vi "Simple Measurement.vi"() -> ()   [LabVIEW 2019]
doc: "Demonstrates how to initialize the bridge, configure measurement parameters, and perform both single and continuous measurements."
uses:
  <vilib>/Utility/file.llb/Write To Spreadsheet File (string).vi
  Andeen-Hagerling 2700A.lvlib
panel:
  in  "Clear":bool
  out "loss graph data":dbl[](array[numeric])
  out "time graph data":timestamp[](array[timestamp])
  out "cap graph data":dbl[](array[numeric])
  out "Measurement Buffer":string[](array[string])
  in  "Save":bool
  in  "cancel measure":bool
  out "Interface Information:Interface Type":u16(ring)=1 items=["GPIB"=1, "VXI"=2, "GPIB-VXI"=3, "Serial"=4, "PXI"=5, "TCPIP"=6, "USB"=7, "FireWire"=9]
  out "V 2":string
  out "Hz 2":string
  out "Capacitance Graph":cluster{timestamp[], dbl[]}(graph)
  out "Loss Graph":cluster{timestamp[], dbl[]}(graph)
  in  "Continuous":bool
  out "bridge error":T1
  out "Bridge Status":string
  out "Error Message":string
  out "V":string
  out "Hz":string
  out "pF":string
  in  "units":i32(ring)=1 items=["NS"=1, "DS"=2, "KO"=3, "GO"=4, "JP"=5]
  out "Applied Voltage":dbl format="%#_10f"
  out "Firmware Revision:":string
  in  "Maximum Applied Voltage":dbl=15.0
  in  "Average\nExponent":i32=4
  in  "Bridge Frequency":dbl=1000.0
  in  "stop":bool
  out "greater than":string
  out "Loss":dbl format="%#_10f"
  out "Measurement Frequency":dbl format="%#_10f"
  out "Capacitance":dbl format="%#_10f"
  out "measurement results":T2 {"Loss" format="%#_10f"; "Capacitance" format="%#_10f"; "Frequency" format="%#_8f"}
  in  "Measure":bool
  # "AH2700A ULTRA-PRECISION CAPACITANCE BRIDGE"
  # "Measurement Parameters"
  # "Measurement Results"
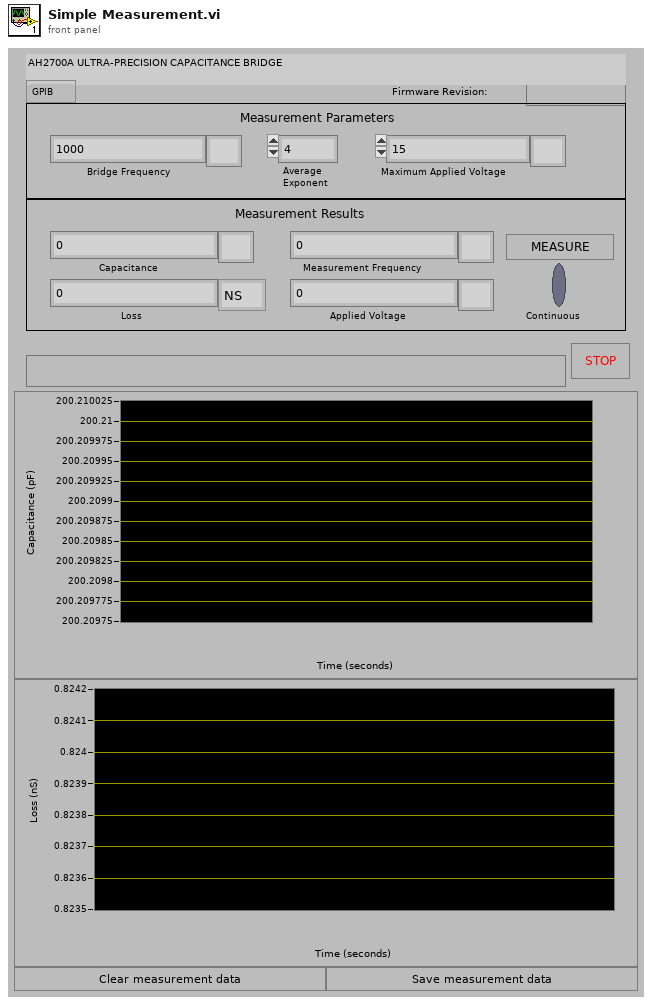
[diagram p1: front panel]
types:
  T1 = cluster{"error message":string, "error code":i32}
  T2 = cluster{"Error":i32, "Frequency":dbl, "Capacitance":dbl, "Loss":dbl, "GreaterThan":bool, "Voltage":dbl}
  T3 = cluster{"Baud Rate":u32, "Parity":u16, "Data Bits":u16, "Stop Bits":u16, "Flow Control":u16}
  T4 = cluster{"error":i32, "frequency":dbl, "capacitance":dbl, "loss":dbl, "greater than":bool, "voltage":dbl}
  T5 = cluster{"time graph data":timestamp[], "cap graph data":dbl[]}
  T6 = cluster{"time graph data":timestamp[], "loss graph data":dbl[]}
  T7 = cluster{"error code":i32, "frequency":dbl, "capacitance":dbl, "loss":dbl, "greater than":bool, "voltage":dbl}
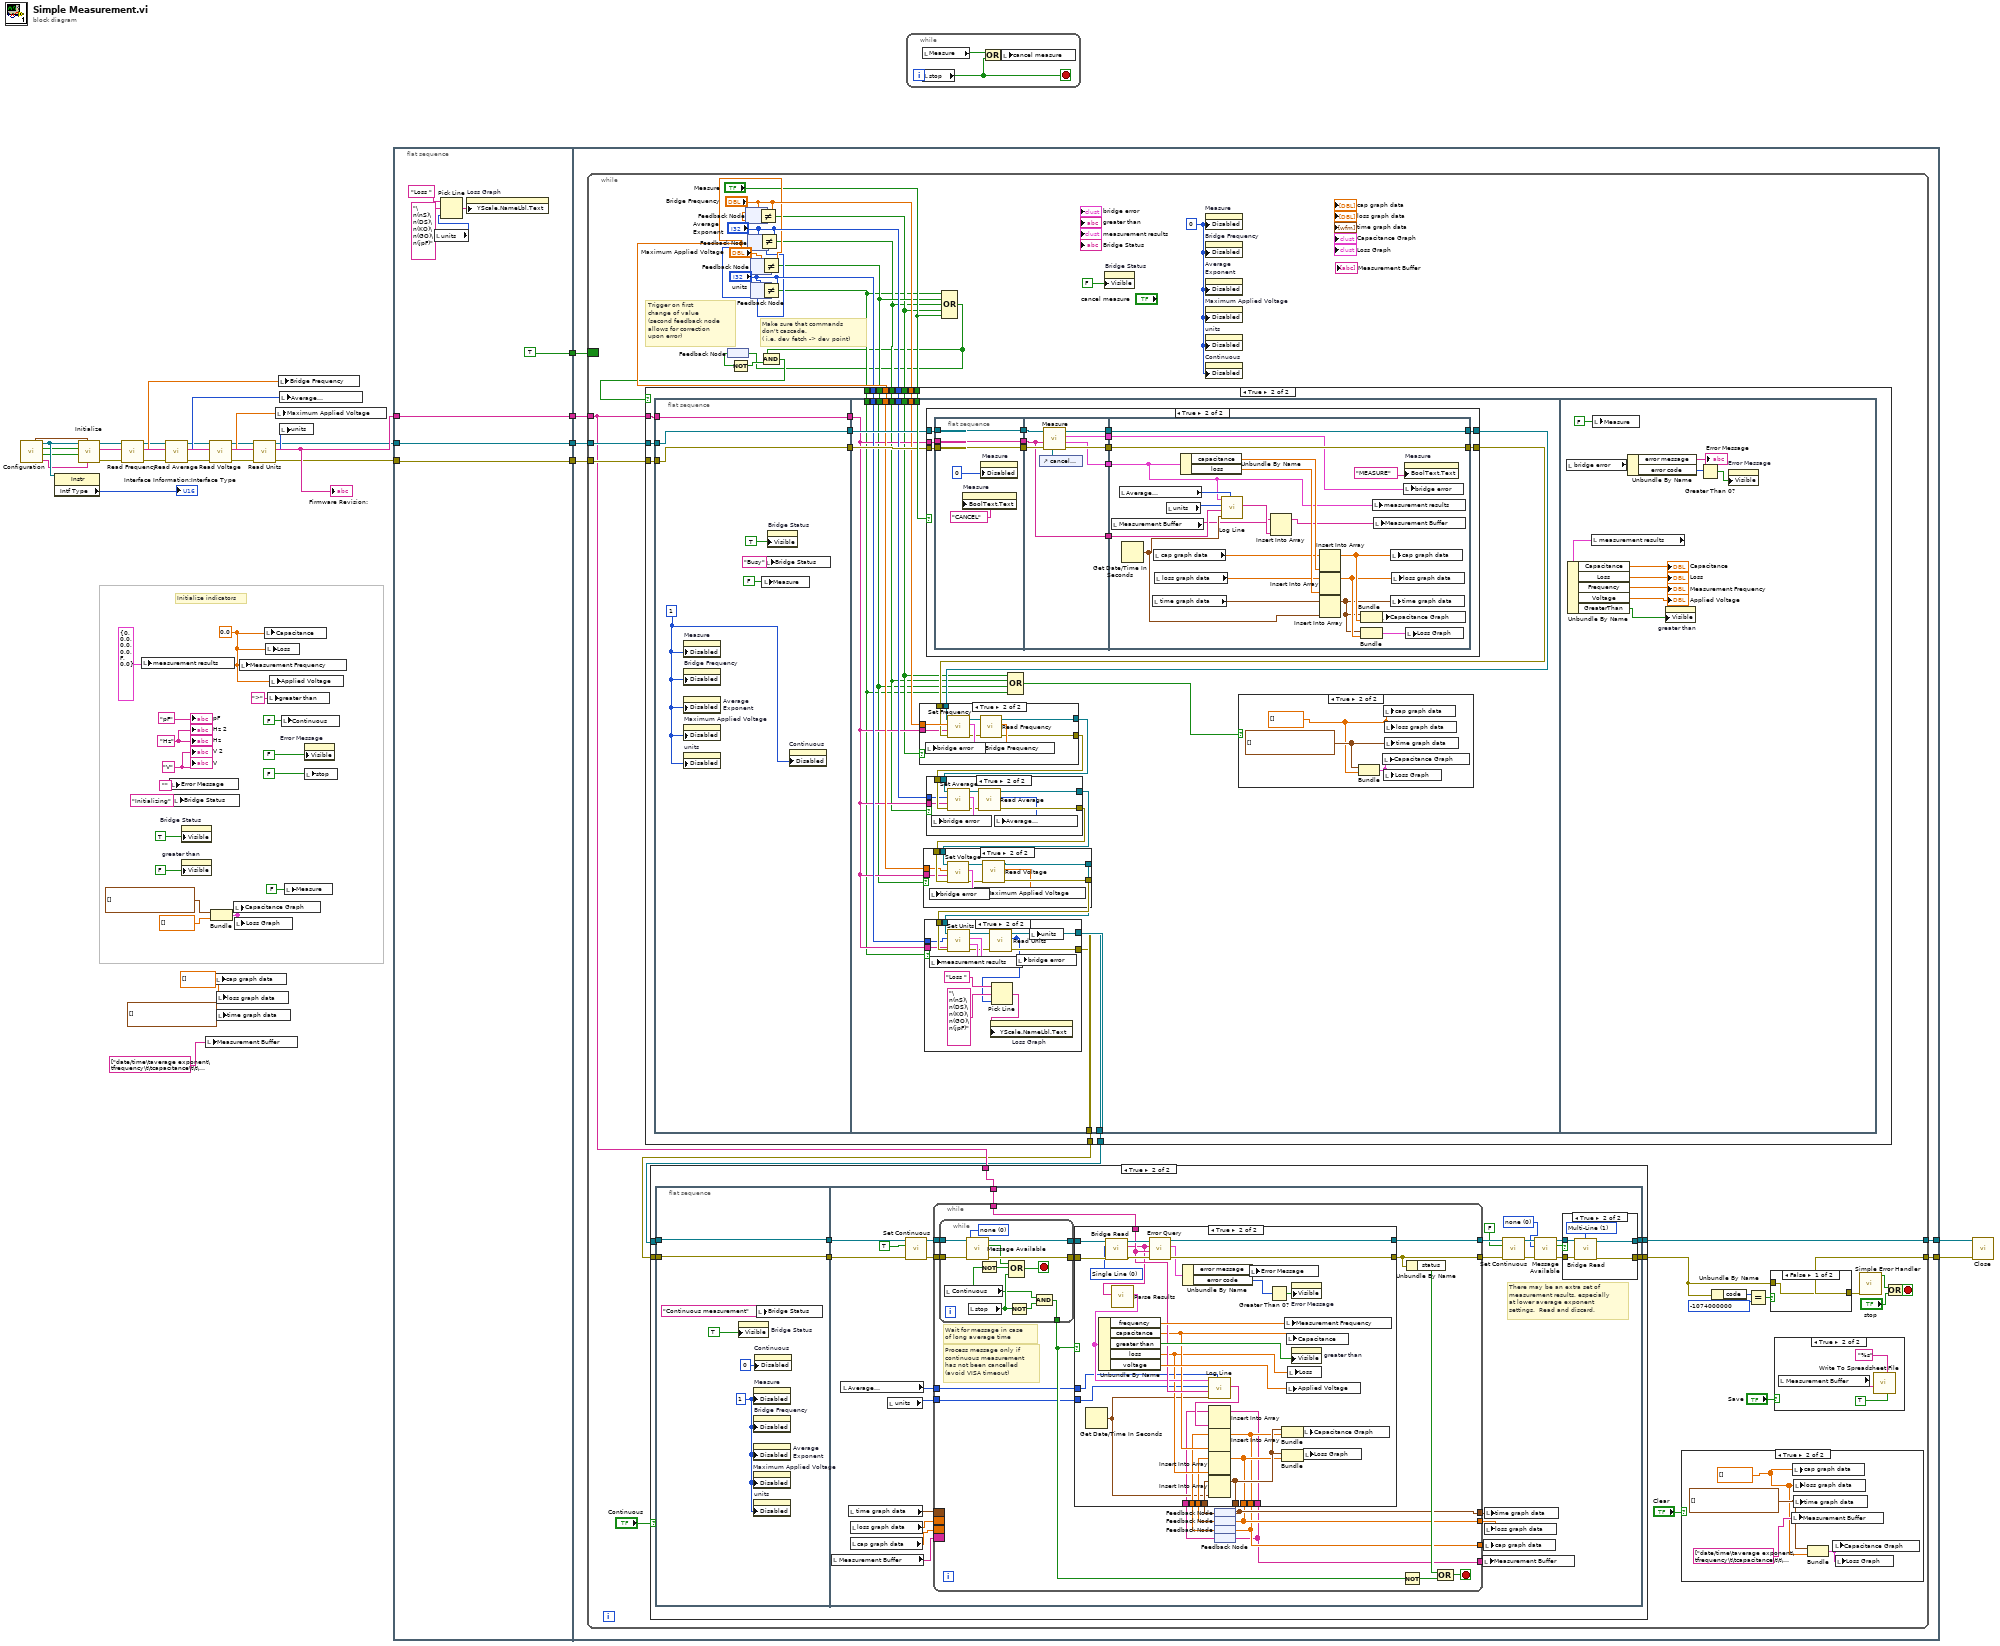
[diagram p0: block diagram]
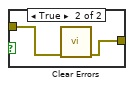
[diagram p14: hidden frame]
diagram:
  w3 = dbl[] [] ("cap graph data")
  w29 = "V" ("V")
  w30 = "Hz" ("Hz")
  w42 = 0.0 ("Capacitance")
  # "Initialize indicators"
  n1 = call "Configuration.vi"() -> ("firmware version"=w6:string, "Reset"=w24:bool, "ID Query"=w7:bool, "VISA resource name out"=w28:refnum<visa-resource-name>, "serial configuration out"=w47:T3)  [unwired: 7 in]
  n2 = property class="Instr"(reference=w28) -> ("Intf Type"=→"Interface Information:Interface Type":u16)  [unwired: 1 in, 2 out]
  n3 = call "Initialize.vi"("firmware revision"=w6, "Serial Configuration"=w47, "Reset (True)"=w24, "ID Query (True)"=w7, "VISA resource name"=w28) -> ("error out"=w10:errorcluster, "firmware revision"=w34:string, "VISA resource name out"=w11:refnum<visa-resource-name>)  [unwired: 4 in]
  "Firmware Revision:" <- w34
  n4 = call "Read Frequency.vi"("error in (no error)"=w10, "VISA resource name"=w11) -> ("error out"=w16:errorcluster, "frequency"=w20:dbl, "VISA resource name out"=w17:refnum<visa-resource-name>)  [unwired: 7 in]
  n5 = local write "measurement results"(T2 {"Error"=0, "Frequency"=0.0, "Capacitance"=0.0, "Loss"=0.0, "GreaterThan"=FALSE, "Voltage"=0.0} ("measurement results")) -> ()
  n6 = call "Read Average.vi"("error in (no error)"=w16, "VISA resource name"=w17) -> ("error out"=w14:errorcluster, "average"=w21:i32, "VISA resource name out"=w15:refnum<visa-resource-name>)  [unwired: 7 in]
  n7 = local write "Error Message"("") -> ()
  n8 = local write "Bridge Status"("Initializing" ("Error Message")) -> ()
  n9 = property on="Bridge Status" class="Str"("Visible"=TRUE) -> ()  [unwired: 2 in, 2 out]
  n10 = property on="greater than" class="Str"("Visible"=FALSE) -> ()  [unwired: 2 in, 2 out]
  n11 = local write "Measurement Buffer"(string[] ["date/time\taverage exponent\tfrequency\t\tcapacitance\t\t\tloss\t\tvoltage\t\terror code\terror message"]) -> ()
  n12 = call "Read Voltage.vi"("error in (no error)"=w14, "VISA resource name"=w15) -> ("error out"=w12:errorcluster, "voltage"=w22:dbl, "VISA resource name out"=w13:refnum<visa-resource-name>)  [unwired: 7 in]
  n13 = Bundle(timestamp[] [], dbl[] []) -> (w31:cluster{timestamp[], dbl[]})  [unwired: 1 in]
  n14 = local write "cap graph data"(w3) -> ()
  n15 = local write "loss graph data"(w3) -> ()
  n16 = local write "time graph data"(timestamp[] [] ("time graph data")) -> ()
  n17 = local write "Capacitance Graph"(w31) -> ()
  n18 = local write "Loss Graph"(w31) -> ()
  n19 = local write "Measurement Frequency"(w42) -> ()
  n20 = call "Read Units.vi"("error in (no error)"=w12, "VISA resource name"=w13) -> ("error out"=w18:errorcluster, "units"=w23:i32, "VISA resource name out"=w19:refnum<visa-resource-name>)  [unwired: 7 in]
  n21 = local write "Capacitance"(w42) -> ()
  n22 = local write "Loss"(w42) -> ()
  n23 = local write "greater than"(">" ("greater than")) -> ()
  n24 = local write "Applied Voltage"(w42) -> ()
  n25 = local write "Maximum Applied Voltage"(w22) -> ()
  n26 = local write "Bridge Frequency"(w20) -> ()
  n27 = local write "Average\nExponent"(w21) -> ()
  n28 = local write "units"(w23) -> ()
  n29 = local write "Continuous"(FALSE ("Continuous")) -> ()
  n30 = local write "Measure"(FALSE ("Measure")) -> ()
  n31 = property on="Error Message" class="Str"("Visible"=FALSE) -> ()  [unwired: 2 in, 2 out]
  n32 = local write "stop"(FALSE ("stop")) -> ()
  n33 = flat-sequence {
    tunnel: w18 -> [w53]
    tunnel: w19 -> [w54]
    tunnel: w34 -> [w55]
    tunnel: [w55] -> w37
    tunnel: [w54] -> w36
    tunnel: [w53] -> w35
    tunnel: [TRUE] -> w26
    tunnel: [w61] -> w45
    tunnel: [w60] -> w44
    tunnel: w37 -> [w59]
    tunnel: w36 -> [w58]
    tunnel: w35 -> [w57]
    tunnel: w26 -> [w56]
    frame #0 {
      n34 = local read "units"() -> (w49:i32)
      n35 = Pick Line(string ("")="Loss ", multi-line string="\n(nS)\n(DS)\n(KO)\n(GO)\n(jpF)", line index=w49) -> (output string=w48:string)
      n36 = property on="Loss Graph" class="XYGraph (strict)"("YScale.NameLbl.Text"=w48) -> ()  [unwired: 2 in, 2 out]
    }
    frame #1 {
      n37 = while {
        tunnel: w58 -> [w98]
        tunnel: w57 -> [w97]
        tunnel: [w93] -> w61
        tunnel: [w75] -> w60
        tunnel: w59 -> [w74]
        border: w56 -> [_]
        stop <- w94 stop-if-true
        w65 = u8 0 ("Disabled")
        # "Trigger on first\nchange of value\n(second feedback node\nallows for correction\nupon error)"
        # "Make sure that commands\ndon't cascade. \n( i.e. dev fetch -> dev point)"
        n38 = feedback #1() -> (w70:bool)
        n39 = Not(x=w70) -> (.not. x?=w71:bool)
        n40 = feedback-in #2("Bridge Frequency") -> ()
        n41 = feedback #2() -> (w83:dbl)  [unwired: 1 in]
        n42 = feedback-in #3("Average\nExponent") -> ()
        n43 = feedback #3() -> (w82:i32)  [unwired: 1 in]
        n44 = feedback-in #4("Maximum Applied Voltage") -> ()
        n45 = feedback #4() -> (w81:dbl)  [unwired: 1 in]
        n46 = feedback-in #5("units") -> ()
        n47 = feedback #5() -> (w80:i32)  [unwired: 1 in]
        n48 = Not Equal?(x="Bridge Frequency", y=w83) -> (x != y?=w68:bool)
        n49 = Not Equal?(x="Average\nExponent", y=w82) -> (x != y?=w67:bool)
        n50 = Not Equal?(x="units", y=w80) -> (x != y?=w66:bool)
        n51 = Not Equal?(x="Maximum Applied Voltage", y=w81) -> (x != y?=w69:bool)
        n52 = Compound Arithmetic op=OR(w66, w69, w67, w68, "Measure") -> (w64:bool)
        n53 = feedback-in #1(w64) -> ()
        n54 = And(x=w64, y=w71) -> (x .and. y?=w78:bool)
        n55 = case shown="True" w78 {
          tunnel: w98 -> [w227 w243]
          tunnel: w97 -> [w228 w242]
          tunnel: "Measure" -> [_ w241]
          tunnel: w68 -> [_ w240]
          tunnel: "Bridge Frequency" -> [_ w239]
          tunnel: "Average\nExponent" -> [_ w238]
          tunnel: w67 -> [_ w237]
          tunnel: "Maximum Applied Voltage" -> [_ w236]
          tunnel: w69 -> [_ w235]
          tunnel: "units" -> [_ w234]
          tunnel: w66 -> [_ w233]
          tunnel: w74 -> [_ w231]
          tunnel: [w227 w230] -> w73
          tunnel: [w228 w229] -> w72
          frame False {
          }
          frame True {
            n56 = flat-sequence {
              tunnel: w242 -> [w251]
              tunnel: w243 -> [w252]
              tunnel: [w252] -> w245
              tunnel: [w251] -> w244
              tunnel: [w249] -> w232
              tunnel: w231 -> [w249]
              tunnel: w241 -> [w275]
              tunnel: w245 -> [w274]
              tunnel: w244 -> [w273]
              tunnel: w240 -> [w256]
              tunnel: w239 -> [w272]
              tunnel: w238 -> [w269]
              tunnel: w237 -> [w255]
              tunnel: w236 -> [w266]
              tunnel: w235 -> [w254]
              tunnel: w234 -> [w262]
              tunnel: w233 -> [w253]
              tunnel: w232 -> [w260]
              tunnel: [w259] -> w230
              tunnel: [w258] -> w229
              frame #0 {
                w247 = u8 1 ("Disabled")
                n57 = property on="Measure" class="Bool (strict)"("Disabled"=w247) -> ()  [unwired: 2 in, 2 out]
                n58 = property on="Bridge Frequency" class="DigNum (strict)"("Disabled"=w247) -> ()  [unwired: 2 in, 2 out]
                n59 = property on="Average\nExponent" class="DigNum (strict)"("Disabled"=w247) -> ()  [unwired: 2 in, 2 out]
                n60 = property on="Maximum Applied Voltage" class="DigNum (strict)"("Disabled"=w247) -> ()  [unwired: 2 in, 2 out]
                n61 = property on="units" class="Ring (strict)"("Disabled"=w247) -> ()  [unwired: 2 in, 2 out]
                n62 = local write "Measure"(FALSE ("Measure")) -> ()
                n63 = local write "Bridge Status"("Busy" ("Bridge Status")) -> ()
                n64 = property on="Bridge Status" class="Str"("Visible"=TRUE) -> ()  [unwired: 2 in, 2 out]
                n65 = property on="Continuous" class="Bool (strict)"("Disabled"=w247) -> ()  [unwired: 2 in, 2 out]
              }
              frame #1 {
                n66 = case shown="True" w275 {
                  tunnel: w274 -> [w332 w345]
                  tunnel: w273 -> [w331 w344]
                  tunnel: [w331 w342] -> w270
                  tunnel: [w332 w343] -> w271
                  tunnel: w260 -> [_ w341]
                  frame False {
                  }
                  frame True {
                    n67 = flat-sequence {
                      tunnel: w341 -> [w348]
                      tunnel: w344 -> [w349]
                      tunnel: w345 -> [w350]
                      tunnel: [w350] -> w340
                      tunnel: [w349] -> w339
                      tunnel: [w348] -> w338
                      tunnel: w340 -> [w358]
                      tunnel: w339 -> [w357]
                      tunnel: w338 -> [w352]
                      tunnel: [w356] -> w337
                      tunnel: [w355] -> w336
                      tunnel: [w353] -> w335
                      tunnel: [w352] -> w334
                      tunnel: [w351] -> w333
                      tunnel: [w379] -> w342
                      tunnel: [w380] -> w343
                      tunnel: w337 -> [w380]
                      tunnel: w336 -> [w379]
                      tunnel: w335 -> [w366]
                      tunnel: w334 -> [w371]
                      tunnel: w333 -> [w367]
                      frame #0 {
                        n68 = property on="Measure" class="Bool (strict)"("BoolText.Text"="CANCEL" ("Boolean Text.Text")) -> ()  [unwired: 2 in, 2 out]
                        n69 = property on="Measure" class="Bool (strict)"("Disabled"=u8 0) -> ()  [unwired: 2 in, 2 out]
                      }
                      frame #1 {
                        n70 = control-ref of="cancel measure"() -> (w354:refnum<vi>)
                        n71 = call "Measure.vi"("cancel refnum"=w354, "error in (no error)"=w357, "firmware revision"=w352, "VISA resource name"=w358) -> ("error out"=w355:errorcluster, "measurement results"=w353:T4, "bridge error"=w351:T1, "VISA resource name out"=w356:refnum<visa-resource-name>)  [unwired: 3 in]
                      }
                      frame #2 {
                        n72 = local read "Measurement Buffer"() -> (w360:string[])
                        n73 = local read "Average\nExponent"() -> (w370:i32)
                        n74 = Get Date/Time In Seconds() -> (seconds since 1Jan1904=w362:timestamp)
                        n75 = local read "time graph data"() -> (w363:timestamp[])
                        n76 = local read "cap graph data"() -> (w365:dbl[])
                        n77 = local read "loss graph data"() -> (w364:dbl[])
                        n78 = local read "units"() -> (w372:i32)
                        n79 = Unbundle By Name(w366) -> ("capacitance"=w369:dbl, "loss"=w368:dbl)
                        n80 = call "Log Line.vi"("average exponent"=w370, "current time"=w362, "firmware revision"=w371, "units"=w372, "measurement results"=w366) -> ("log line"=w361:string)  [unwired: 6 in]
                        n81 = Insert Into Array(array=w360, new element=w361) -> (w359:string[])  [unwired: 1 in]
                        n82 = Insert Into Array(array=w365, new element=w369) -> (w375:dbl[])  [unwired: 1 in]
                        n83 = Insert Into Array(array=w364, new element=w368) -> (w374:dbl[])  [unwired: 1 in]
                        n84 = Insert Into Array(array=w363, new element=w362) -> (w373:timestamp[])  [unwired: 1 in]
                        n85 = Bundle("time graph data"=w373, "cap graph data"=w375) -> (w377:T5)  [unwired: 1 in]
                        n86 = Bundle("time graph data"=w373, "loss graph data"=w374) -> (w376:T6)  [unwired: 1 in]
                        n87 = local write "measurement results"(w366) -> ()
                        n88 = local write "Measurement Buffer"(w359) -> ()
                        n89 = local write "Capacitance Graph"(w377) -> ()
                        n90 = local write "cap graph data"(w375) -> ()
                        n91 = local write "time graph data"(w373) -> ()
                        n92 = local write "loss graph data"(w374) -> ()
                        n93 = local write "bridge error"(w367) -> ()
                        n94 = property on="Measure" class="Bool (strict)"("BoolText.Text"="MEASURE" ("Boolean Text.Text")) -> ()  [unwired: 2 in, 2 out]
                        n95 = local write "Loss Graph"(w376) -> ()
                      }
                    }
                  }
                }
                n96 = case shown="True" w256 {
                  tunnel: w272 -> [_ w330]
                  tunnel: w271 -> [w320 w329]
                  tunnel: w270 -> [w319 w328]
                  tunnel: w260 -> [_ w327]
                  tunnel: [w320 w322] -> w268
                  tunnel: [w319 w321] -> w267
                  frame False {
                  }
                  frame True {
                    n97 = call "Set Frequency.vi"("error in (no error)"=w328, "firmware revision"=w327, "frequency (1000)"=w330, "VISA resource name"=w329) -> ("error out"=w324:errorcluster, "bridge error"=w326:T1, "VISA resource name out"=w325:refnum<visa-resource-name>)  [unwired: 5 in]
                    n98 = local write "bridge error"(w326) -> ()
                    n99 = call "Read Frequency.vi"("error in (no error)"=w324, "VISA resource name"=w325) -> ("error out"=w321:errorcluster, "frequency"=w323:dbl, "VISA resource name out"=w322:refnum<visa-resource-name>)  [unwired: 7 in]
                    n100 = local write "Bridge Frequency"(w323) -> ()
                  }
                }
                n101 = case shown="True" w255 {
                  tunnel: w268 -> [w308 w318]
                  tunnel: w267 -> [w307 w317]
                  tunnel: [w308 w310] -> w264
                  tunnel: [w307 w312] -> w265
                  tunnel: w269 -> [_ w316]
                  tunnel: w260 -> [_ w315]
                  frame False {
                  }
                  frame True {
                    n102 = call "Set Average.vi"("error in (no error)"=w317, "firmware revision"=w315, "average (4)"=w316, "VISA resource name"=w318) -> ("error out"=w313:errorcluster, "bridge error"=w314:T1, "VISA resource name out"=w311:refnum<visa-resource-name>)  [unwired: 5 in]
                    n103 = local write "bridge error"(w314) -> ()
                    n104 = call "Read Average.vi"("error in (no error)"=w313, "VISA resource name"=w311) -> ("error out"=w312:errorcluster, "average"=w309:i32, "VISA resource name out"=w310:refnum<visa-resource-name>)  [unwired: 7 in]
                    n105 = local write "Average\nExponent"(w309) -> ()
                  }
                }
                n106 = case shown="True" w254 {
                  tunnel: w264 -> [w296 w306]
                  tunnel: w265 -> [w295 w305]
                  tunnel: [w296 w300] -> w261
                  tunnel: [w295 w298] -> w263
                  tunnel: w260 -> [_ w304]
                  tunnel: w266 -> [_ w303]
                  frame False {
                  }
                  frame True {
                    n107 = call "Set Voltage.vi"("error in (no error)"=w305, "firmware revision"=w304, "voltage (15)"=w303, "VISA resource name"=w306) -> ("error out"=w299:errorcluster, "bridge error"=w302:T1, "VISA resource name out"=w301:refnum<visa-resource-name>)  [unwired: 5 in]
                    n108 = local write "bridge error"(w302) -> ()
                    n109 = call "Read Voltage.vi"("error in (no error)"=w299, "VISA resource name"=w301) -> ("error out"=w298:errorcluster, "voltage"=w297:dbl, "VISA resource name out"=w300:refnum<visa-resource-name>)  [unwired: 7 in]
                    n110 = local write "Maximum Applied Voltage"(w297) -> ()
                  }
                }
                n111 = case shown="True" w253 {
                  tunnel: w261 -> [w280 w294]
                  tunnel: w263 -> [w279 w293]
                  tunnel: [w280 w285] -> w259
                  tunnel: [w279 w287] -> w258
                  tunnel: w260 -> [_ w292]
                  tunnel: w262 -> [_ w291]
                  frame False {
                  }
                  frame True {
                    n112 = call "Set Units.vi"("error in (no error)"=w293, "firmware revision"=w292, "units (NS)"=w291, "VISA resource name"=w294) -> ("error out"=w288:errorcluster, "measurement results"=w290:T2, "bridge error"=w289:T1, "VISA resource name out"=w286:refnum<visa-resource-name>)  [unwired: 4 in]
                    n113 = local write "measurement results"(w290) -> ()
                    n114 = call "Read Units.vi"("error in (no error)"=w288, "VISA resource name"=w286) -> ("error out"=w287:errorcluster, "units"=w282:i32, "VISA resource name out"=w285:refnum<visa-resource-name>)  [unwired: 7 in]
                    n115 = Pick Line(string ("")="Loss ", multi-line string="\n(nS)\n(DS)\n(KO)\n(GO)\n(jpF)", line index=w282) -> (output string=w281:string)
                    n116 = property on="Loss Graph" class="XYGraph (strict)"("YScale.NameLbl.Text"=w281) -> ()  [unwired: 2 in, 2 out]
                    n117 = local write "bridge error"(w289) -> ()
                    n118 = local write "units"(w282) -> ()
                  }
                }
                n119 = Compound Arithmetic op=OR(w256, w255, w254, w253) -> (w257:bool)
                n120 = case shown="True" w257 {
                  frame False {
                  }
                  frame True {
                    w276 = dbl[] []
                    w277 = timestamp[] [] ("time graph data")
                    n121 = Bundle("time graph data"=w277, w276) -> (w278:cluster{"time graph data":timestamp[], dbl[]})  [unwired: 1 in]
                    n122 = local write "Capacitance Graph"(w278) -> ()
                    n123 = local write "cap graph data"(w276) -> ()
                    n124 = local write "Loss Graph"(w278) -> ()
                    n125 = local write "loss graph data"(w276) -> ()
                    n126 = local write "time graph data"(w277) -> ()
                  }
                }
              }
              frame #2 {
                n127 = local read "bridge error"() -> (w390:T1)
                n128 = local read "measurement results"() -> (w389:T2)
                n129 = Unbundle By Name(w389) -> ("Capacitance"=→"Capacitance":dbl, "Loss"=→"Loss":dbl, "Frequency"=→"Measurement Frequency":dbl, "Voltage"=→"Applied Voltage":dbl, "GreaterThan"=w381:bool)
                n130 = local write "Measure"(FALSE ("Measure")) -> ()
                n131 = Unbundle By Name(w390) -> ("error message"=→"Error Message":string, "error code"=w384:i32)
                n132 = property on="greater than" class="Str"("Visible"=w381) -> ()  [unwired: 2 in, 2 out]
                n133 = Greater Than 0?(x=w384) -> (x > 0?=w383:bool)
                n134 = property on="Error Message" class="Str"("Visible"=w383) -> ()  [unwired: 2 in, 2 out]
              }
            }
          }
        }
        n135 = case shown="True" "Continuous" {
          tunnel: w73 -> [w107 w114]
          tunnel: w72 -> [w106 w113]
          tunnel: [w106 w112] -> w76
          tunnel: [w107 w111] -> w75
          tunnel: w74 -> [_ w110]
          frame False {
          }
          frame True {
            n136 = flat-sequence {
              tunnel: w113 -> [w119]
              tunnel: w114 -> [w120]
              tunnel: [w120] -> w109
              tunnel: [w119] -> w108
              tunnel: w110 -> [w139]
              tunnel: w109 -> [w142]
              tunnel: w108 -> [w141]
              tunnel: [w132] -> w112
              tunnel: [w133] -> w111
              frame #0 {
                w116 = u8 1 ("Disabled")
                n137 = property on="Bridge Status" class="Str"("Visible"=TRUE) -> ()  [unwired: 2 in, 2 out]
                n138 = property on="Measure" class="Bool (strict)"("Disabled"=w116) -> ()  [unwired: 2 in, 2 out]
                n139 = property on="Bridge Frequency" class="DigNum (strict)"("Disabled"=w116) -> ()  [unwired: 2 in, 2 out]
                n140 = property on="Average\nExponent" class="DigNum (strict)"("Disabled"=w116) -> ()  [unwired: 2 in, 2 out]
                n141 = property on="Maximum Applied Voltage" class="DigNum (strict)"("Disabled"=w116) -> ()  [unwired: 2 in, 2 out]
                n142 = property on="units" class="Ring (strict)"("Disabled"=w116) -> ()  [unwired: 2 in, 2 out]
                n143 = property on="Continuous" class="Bool (strict)"("Disabled"=u8 0) -> ()  [unwired: 2 in, 2 out]
                n144 = local write "Bridge Status"("Continuous measurement" ("Bridge Status")) -> ()
              }
              frame #1 {
                w136 = u16 0 items=["none", "error check", "multiline read", "infinite"] ("delay")
                # "There may be an extra set of\nmeasurement results, especially\nat lower average exponent \nsettings.  Read and discard."
                n145 = local read "Measurement Buffer"() -> (w124:string[])
                n146 = local read "Average\nExponent"() -> (w122:i32)
                n147 = local read "time graph data"() -> (w130:timestamp[])
                n148 = local read "loss graph data"() -> (w129:dbl[])
                n149 = local read "cap graph data"() -> (w128:dbl[])
                n150 = local read "units"() -> (w121:i32)
                n151 = call "Set Continuous.vi"("error in (no error)"=w141, "continuous mode (F)"=TRUE, "VISA resource name"=w142) -> ("error out"=w146:errorcluster, "VISA resource name out"=w145:refnum<visa-resource-name>)  [unwired: 7 in]
                n152 = while {
                  tunnel: w146 -> [w172]
                  tunnel: w145 -> [w165]
                  tunnel: [w175] -> w144
                  tunnel: [w169] -> w143
                  tunnel: w139 -> [w174]
                  tunnel: [w161] -> w127
                  tunnel: [w160] -> w126
                  tunnel: [w159] -> w125
                  tunnel: [w157] -> w123
                  tunnel: w122 -> [w156]
                  tunnel: w121 -> [w155]
                  border: w130 -> [_]
                  border: w129 -> [_]
                  border: w128 -> [_]
                  border: w124 -> [_]
                  stop <- w173 stop-if-true
                  # "Process message only if\ncontinuous measurement\nhas not been cancelled\n(avoid VISA timeout)"
                  # "Wait for message in case\nof long average time"
                  n153 = while {
                    tunnel: w165 -> [w226]
                    tunnel: w172 -> [w225]
                    tunnel: [w224] -> w170
                    tunnel: [w223] -> w171
                    tunnel: [w215] -> w166
                    stop <- w220 stop-if-true
                    w219 = u16 0 items=["none", "error check", "multiline read", "infinite"] ("delay")
                    n154 = local read "Continuous"() -> (w217:bool)
                    n155 = call "Message Available.vi"("error in (no error)"=w225, "delay"=w219, "VISA resource name"=w226) -> ("error out"=w224:errorcluster, "message available"=w221:bool, "VISA resource name out"=w223:refnum<visa-resource-name>)  [unwired: 6 in]
                    n156 = local read "stop"() -> (w218:bool)
                    n157 = Not(x=w217) -> (.not. x?=w222:bool)
                    n158 = Compound Arithmetic op=OR(w221, w222, w218) -> (w220:bool)
                    n159 = Not(x=w218) -> (.not. x?=w216:bool)
                    n160 = Compound Arithmetic op=AND(w217, w216) -> (w215:bool)
                  }
                  n161 = feedback #6() -> (w164:timestamp[])
                  n162 = feedback #7() -> (w163:dbl[])
                  n163 = feedback #8() -> (w162:dbl[])
                  n164 = feedback #9() -> (w158:string[])
                  n165 = case shown="True" w166 {
                    tunnel: [w181 w214] -> w175
                    tunnel: [w180 w213] -> w169
                    tunnel: w174 -> [_ w200]
                    tunnel: w171 -> [w181 w210]
                    tunnel: w170 -> [w180 w211]
                    tunnel: [w179 w193] -> w161
                    tunnel: [w178 w192] -> w160
                    tunnel: [w177 w191] -> w159
                    tunnel: w164 -> [w179 w190]
                    tunnel: w163 -> [w178 w189]
                    tunnel: w162 -> [w177 w188]
                    tunnel: [w176 w186] -> w157
                    tunnel: w158 -> [w176 w184]
                    tunnel: w156 -> [_ w183]
                    tunnel: w155 -> [_ w182]
                    frame False {
                    }
                    frame True {
                      w207 = u16 0 items=["Single Line", "Multi-Line"] ("Multiline")
                      n166 = Get Date/Time In Seconds() -> (seconds since 1Jan1904=w187:timestamp)
                      n167 = call "Bridge Read.vi"("error in (no error)"=w211, "multiline"=w207, "VISA resource name"=w210) -> ("error out"=w208:errorcluster, "read buffer"=w199:string, "VISA resource name out"=w209:refnum<visa-resource-name>)  [unwired: 6 in]
                      n168 = call "Parse Results.vi"("measurement line"=w199) -> ("measurement results"=w197:T7)  [unwired: 9 in]
                      n169 = Unbundle By Name(w197) -> ("frequency"=w204:dbl, "capacitance"=w198:dbl, "greater than"=w201:bool, "loss"=w196:dbl, "voltage"=w202:dbl)
                      n170 = call "Error Query.vi"("error in (no error)"=w208, "firmware revision"=w200, "measurement line"=w199, "VISA resource name"=w209) -> ("error out"=w213:errorcluster, "bridge error"=w212:T1, "VISA resource name out"=w214:refnum<visa-resource-name>)  [unwired: 5 in]
                      n171 = Unbundle By Name(w212) -> ("error message"=w203:string, "error code"=w206:i32)
                      n172 = call "Log Line.vi"("average exponent"=w183, "current time"=w187, "firmware revision"=w200, "units"=w182, "measurement results"=w197) -> ("log line"=w185:string)  [unwired: 6 in]
                      n173 = Insert Into Array(array=w184, new element=w185) -> (w186:string[])  [unwired: 1 in]
                      n174 = Insert Into Array(array=w188, new element=w198) -> (w191:dbl[])  [unwired: 1 in]
                      n175 = Insert Into Array(array=w189, new element=w196) -> (w192:dbl[])  [unwired: 1 in]
                      n176 = Insert Into Array(array=w190, new element=w187) -> (w193:timestamp[])  [unwired: 1 in]
                      n177 = local write "Error Message"(w203) -> ()
                      n178 = Greater Than 0?(x=w206) -> (x > 0?=w205:bool)
                      n179 = Bundle("time graph data"=w193, "cap graph data"=w191) -> (w195:T5)  [unwired: 1 in]
                      n180 = Bundle("time graph data"=w193, "loss graph data"=w192) -> (w194:T6)  [unwired: 1 in]
                      n181 = local write "Measurement Frequency"(w204) -> ()
                      n182 = local write "Capacitance"(w198) -> ()
                      n183 = local write "Applied Voltage"(w202) -> ()
                      n184 = local write "Loss"(w196) -> ()
                      n185 = property on="greater than" class="Str"("Visible"=w201) -> ()  [unwired: 2 in, 2 out]
                      n186 = property on="Error Message" class="Str"("Visible"=w205) -> ()  [unwired: 2 in, 2 out]
                      n187 = local write "Capacitance Graph"(w195) -> ()
                      n188 = local write "Loss Graph"(w194) -> ()
                    }
                  }
                  n189 = feedback-in #6(w161) -> ()
                  n190 = feedback-in #7(w160) -> ()
                  n191 = feedback-in #8(w159) -> ()
                  n192 = feedback-in #9(w157) -> ()
                  n193 = Not(x=w166) -> (.not. x?=w168:bool)
                  n194 = Unbundle By Name(w169) -> ("status"=w167:bool)
                  n195 = Compound Arithmetic op=OR(w167, w168) -> (w173:bool)
                }
                n196 = local write "Measurement Buffer"(w123) -> ()
                n197 = local write "cap graph data"(w125) -> ()
                n198 = local write "time graph data"(w127) -> ()
                n199 = local write "loss graph data"(w126) -> ()
                n200 = call "Set Continuous.vi"("error in (no error)"=w143, "continuous mode (F)"=FALSE, "VISA resource name"=w144) -> ("error out"=w137:errorcluster, "VISA resource name out"=w138:refnum<visa-resource-name>)  [unwired: 7 in]
                n201 = call "Message Available.vi"("error in (no error)"=w137, "delay"=w136, "VISA resource name"=w138) -> ("error out"=w134:errorcluster, "message available"=w131:bool, "VISA resource name out"=w135:refnum<visa-resource-name>)  [unwired: 6 in]
                n202 = case shown="True" w131 {
                  tunnel: w135 -> [w149 w153]
                  tunnel: w134 -> [w148 w152]
                  tunnel: [w149 w151] -> w133
                  tunnel: [w148 w150] -> w132
                  frame False {
                  }
                  frame True {
                    w154 = u16 1 items=["Single Line", "Multi-Line"] ("Multiline")
                    n203 = call "Bridge Read.vi"("error in (no error)"=w152, "multiline"=w154, "VISA resource name"=w153) -> ("error out"=w150:errorcluster, "VISA resource name out"=w151:refnum<visa-resource-name>)  [unwired: 6 in, 1 out]
                  }
                }
              }
            }
          }
        }
        n204 = property on="Bridge Status" class="Str"("Visible"=FALSE) -> ()  [unwired: 2 in, 2 out]
        n205 = property on="Measure" class="Bool (strict)"("Disabled"=w65) -> ()  [unwired: 2 in, 2 out]
        n206 = property on="Bridge Frequency" class="DigNum (strict)"("Disabled"=w65) -> ()  [unwired: 2 in, 2 out]
        n207 = property on="Average\nExponent" class="DigNum (strict)"("Disabled"=w65) -> ()  [unwired: 2 in, 2 out]
        n208 = property on="Maximum Applied Voltage" class="DigNum (strict)"("Disabled"=w65) -> ()  [unwired: 2 in, 2 out]
        n209 = property on="units" class="Ring (strict)"("Disabled"=w65) -> ()  [unwired: 2 in, 2 out]
        n210 = property on="Continuous" class="Bool (strict)"("Disabled"=w65) -> ()  [unwired: 2 in, 2 out]
        n211 = case shown="True" "Clear" {
          frame False {
          }
          frame True {
            w99 = dbl[] []
            w102 = timestamp[] [] ("time graph data")
            n212 = local write "Measurement Buffer"(string[] ["date/time\taverage exponent\tfrequency\t\tcapacitance\t\t\tloss\t\tvoltage\t\terror code\terror message"]) -> ()
            n213 = local write "cap graph data"(w99) -> ()
            n214 = local write "loss graph data"(w99) -> ()
            n215 = local write "time graph data"(w102) -> ()
            n216 = Bundle("time graph data"=w102, w99) -> (w101:cluster{"time graph data":timestamp[], dbl[]})  [unwired: 1 in]
            n217 = local write "Capacitance Graph"(w101) -> ()
            n218 = local write "Loss Graph"(w101) -> ()
          }
        }
        n219 = Unbundle By Name(w76) -> ("code"=w88:i32)
        n220 = Equal?(x=w88, y=-1074000000 ("Code")) -> (x = y?=w86:bool)
        n221 = case shown="False" w86 {
          tunnel: w76 -> [w392 w394]
          tunnel: [w392 w393] -> w85
          frame False {
          }
          frame True {
            n222 = call <vilib>:"Clear Errors.vi"("error in (no error)"=w394) -> ("error out"=w393:errorcluster)  [unwired: 5 in, 1 out]
          }
        }
        n223 = case shown="True" "Save" {
          frame False {
          }
          frame True {
            n224 = local read "Measurement Buffer"() -> (w103:string[])
            n225 = call-poly <vilib>:"Write To Spreadsheet File.vi"("transpose? (no:F)"=TRUE, "format (%s)"="%s", "1D data"=w103) -> ()  [unwired: 5 in, 1 out]
          }
        }
        n226 = call <vilib>:"Simple Error Handler.vi"("error in (no error)"=w85) -> ("error?"=w96:bool, "error out"=w93:errorcluster)  [unwired: 4 in, 3 out]
        n227 = Or(x=w96, y="stop") -> (x .or. y?=w94:bool)
      }
    }
  }
  n228 = while {
    stop <- w396 stop-if-true
    n229 = local read "Measure"() -> (w395:bool)
    n230 = local read "stop"() -> (w396:bool)
    n231 = Or(x=w395, y=w396) -> (x .or. y?=w397:bool)
    n232 = local write "cancel measure"(w397) -> ()
  }
  n233 = call "Close.vi"("error in (no error)"=w45, "VISA resource name"=w44) -> ()  [unwired: 9 in, 1 out]
  "pF" <- "pF" ("pF")
  "Hz" <- w30
  "V" <- w29
  "Hz 2" <- w30
  "V 2" <- w29
